vi "close references.vi"(7 "Open Front Panel":bool, 8 "error in":errorcluster, 11 "initialized references":T1[](array[typedef])) -> (0 "error out":errorcluster)   [LabVIEW 2013, in "data interface script.lvlib"]
uses:
  data interface script.lvlib
  Controls/initialized references.ctl
  Controls/interface VI type.ctl
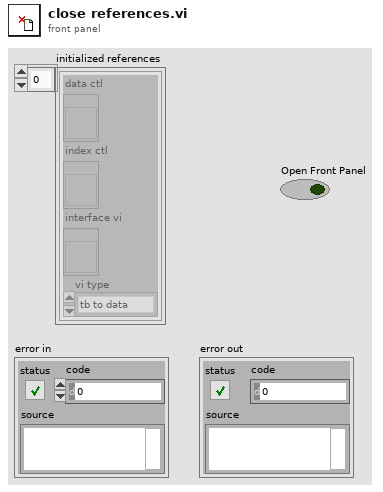
[diagram p1: front panel]
types:
  T1 = typedef "data interface script.lvlib/initialized references.ctl" = cluster{"data ctl":refnum<vi>, "index ctl":refnum<vi>, "interface vi":refnum<vi>, "vi type":T2}
  T2 = typedef "data interface script.lvlib/interface VI type.ctl" = enum16{"tb to data", "data to tb"}
  T3 = enum32{"Invalid", "Standard", "Closed", "Hidden", "Minimized", "Maximized"}
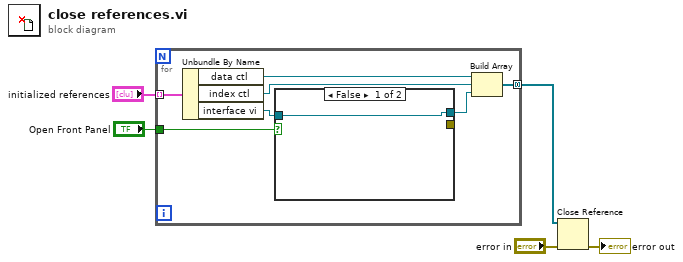
[diagram p0: block diagram]
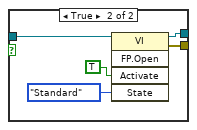
[diagram p2: hidden frame]
diagram:
  n1 = for {
    tunnel: "initialized references" -> [w12] mode=indexing
    tunnel: [w9] -> w2 mode=concatenating
    tunnel: "Open Front Panel" -> [w8]
    n2 = Unbundle By Name(w12) -> ("data ctl"=w10:refnum<vi>, "index ctl"=w11:refnum<vi>, "interface vi"=w7:refnum<vi>)
    n3 = case shown="False" w8 {
      tunnel: w7 -> [w13 w18]
      tunnel: [_ w17] -> _
      tunnel: [w13 w14] -> w6
      frame False {
      }
      frame True {
        n4 = invoke class="VI" method="FP.Open"(reference=w18, "Activate"=TRUE ("Activate?"), "State"=T3."Standard") -> (reference out=w14:refnum<vi>, error out=w17:errorcluster)  [unwired: 2 in, 3 out]
      }
    }
    n5 = Build Array(w10, w11, w6) -> (w9:refnum<vi>[])
  }
  n6 = Close Reference(reference=w2, error in (no error)="error in") -> (error out=→"error out":errorcluster)
